vi "GPIB with VISA functions.vi"() -> ()   [LabVIEW 2020]
doc: "This example requires NI-488.2 and NI-VISA to be installed on the system. The example shows how to communicate with a GPIB instrument using VISA reads, writes, and formatting functions on the returned data. This example will work using an NI Instrument Simulator or other instrument that has similar behavior."
uses:
  <vilib>/Utility/file.llb/Write Delimited Spreadsheet (DBL).vi
  <vilib>/Analysis/NI_AALBase.lvlib
panel:
  out "Acquisition Progress":u8(slide) scale=0.0..100.0
  out "Instrument ID Response":string
  out "Current Time":timestamp
  out "XY Graph":cluster{timestamp[], dbl[]}(graph)
  out "Status Window":string
  out "Tstamp Array":timestamp[](array[timestamp])
  out "FILE WRITE":bool
  out "FILE OPEN":bool
  out "VISA OPEN":bool
  out "SAMPLE":bool
  out "Output Timestamp":timestamp[](array[timestamp])
  in  "Cancel Plot Button":bool caption="Plot Button"
  in  "EXIT":bool caption="Plot Button"
  out "Histogram Graph":T1(graph)
  out "AVG":dbl format="%^.7e"
  out "Units Display":string="VDC"
  out "LCDString":string
  in  "Plot Button":bool
  in  "INSTRUMENT MODE":T2
  out "P-P":dbl format="%^.7e"
  out "MNIDX":i32 format="%#.0f"
  out "MIN":dbl format="%^.7e"
  out "MXIDX":i32 format="%#.0f"
  out "MAX":dbl format="%^.7e"
  out "Output Value Array":dbl[](array[numeric]) format="%^#_8e"
  out "Data Array":dbl[](array[numeric]) format="%^_9e"
  out "ET":dbl format="%<%H:%M:%S%2u>t"
  out "ERROR":bool
  out "ACTIVE CONNECTION":bool
  out "UI Title String":string="IDEwerks IEE488 DataAcquisition/Logging Module" caption="String"
  in  "SETUP PARAMETERS":T3={"Samples"=1024, "NPLC"=10.0, "Digits"=7, "Auto-Zero"="ON", "Auto-Range"="ON", "ACAL on Scan"="ENABLED", "Display"="TEST IN PROGRESS", "Fixed-Z"="OFF", "Man-Range"="OFF", "Panel Lock"="OFF", "Logging"="POST SCAN", "Export Type"=""} {"Digits" min=4 max=8}
  out "SAM":i32
  out "Waveform Chart":waveform(dbl)(graph)
  out "error out":errorcluster
  out "VAL":dbl format="%.7e"
  in  "VISA GPIB Resource":refnum<visa-resource-name>="GPIB0::22::INSTR"
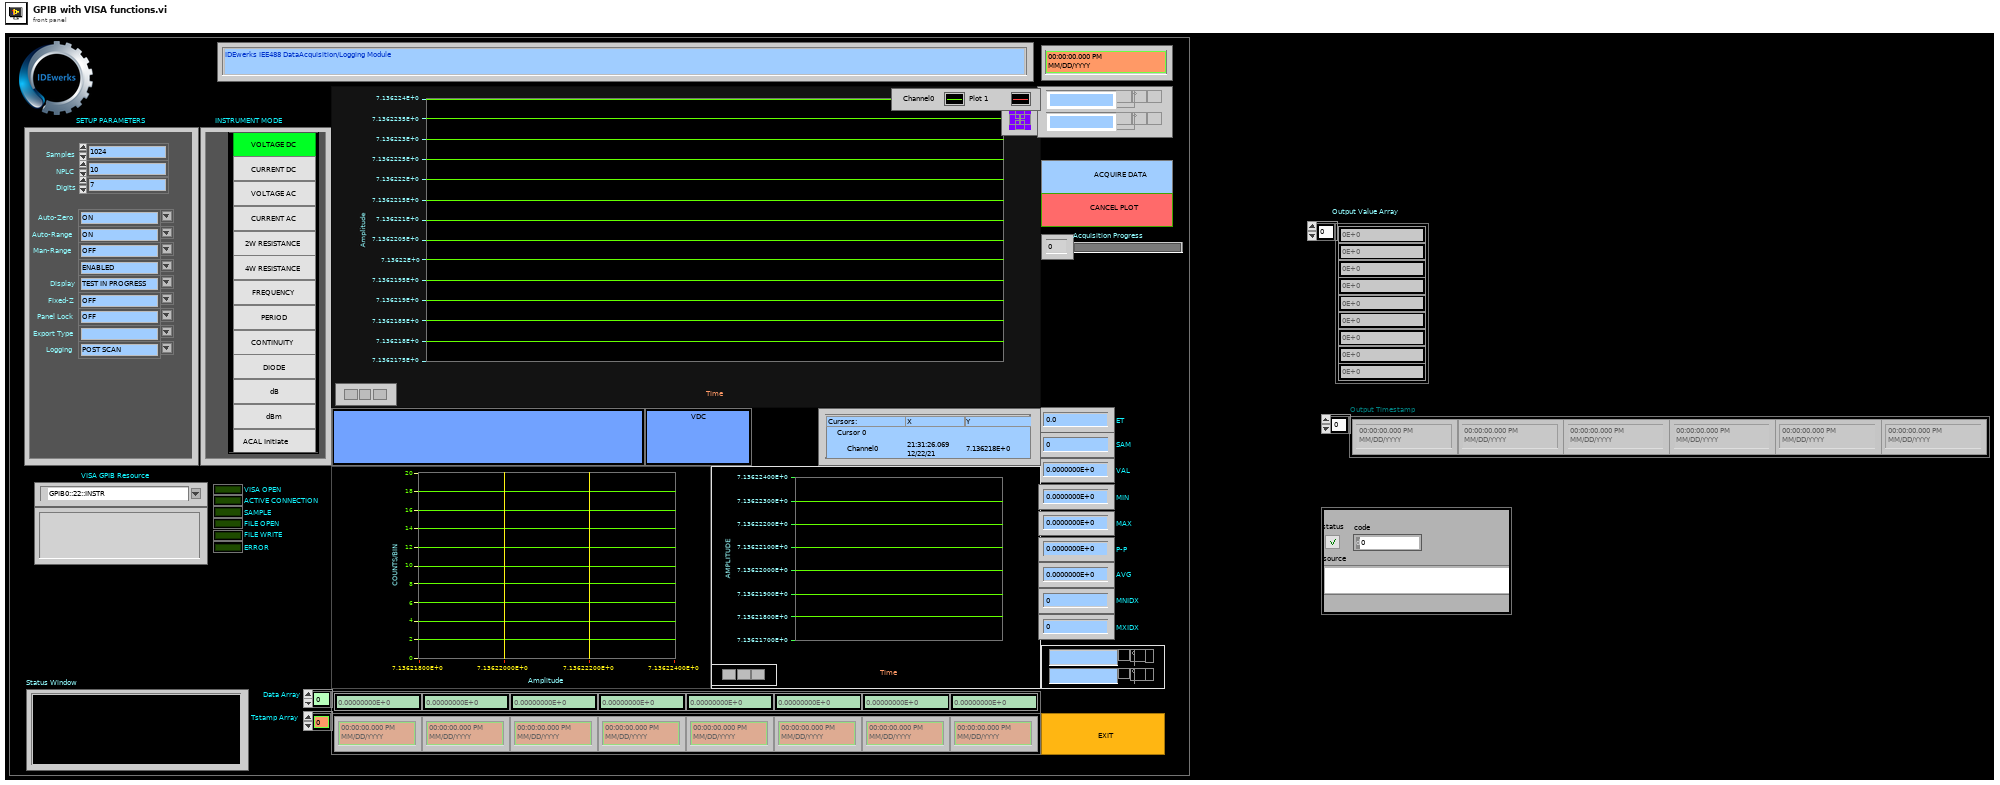
[diagram p1: front panel]
types:
  T1 = cluster{"X Values":dbl[], "Histogram: h(x)":i32[]}
  T2 = cluster{"Radio Buttons":enum32{"VDC Select Button", "IDC Select Button", "VAC Select Button", "IAC Select Button", "2WR Select Button", "4W Res Select Button", "Freq Select Button", "Period Select Button", "Continuity Select Button", "Diode Select Button", "dB Select Button", "dBm Select Button", "ACAL Select Button"}}
  T3 = cluster{"Samples":i32, "NPLC":dbl, "Digits":i32, "Auto-Zero":string, "Auto-Range":string, "ACAL on Scan":string, "Display":string, "Fixed-Z":string, "Man-Range":string, "Panel Lock":string, "Logging":string, "Export Type":string}
  T4 = enum32{"VDC Select Button", "IDC Select Button", "VAC Select Button", "IAC Select Button", "2WR Select Button", "4W Res Select Button", "Freq Select Button", "Period Select Button", "Continuity Select Button", "Diode Select Button", "dB Select Button", "dBm Select Button", "ACAL Select Button"}
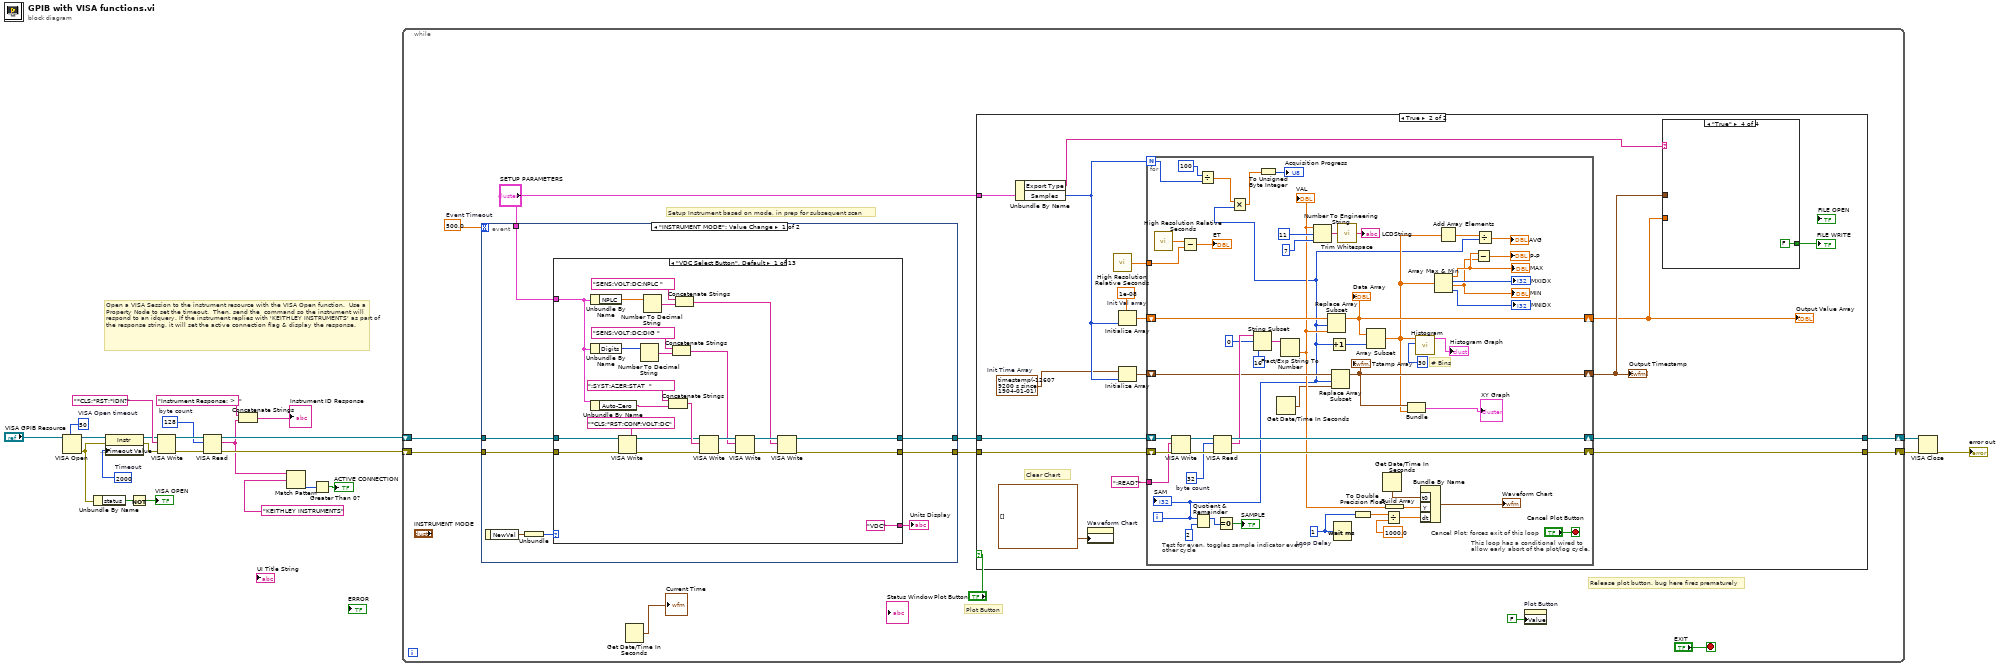
[diagram p0: block diagram]
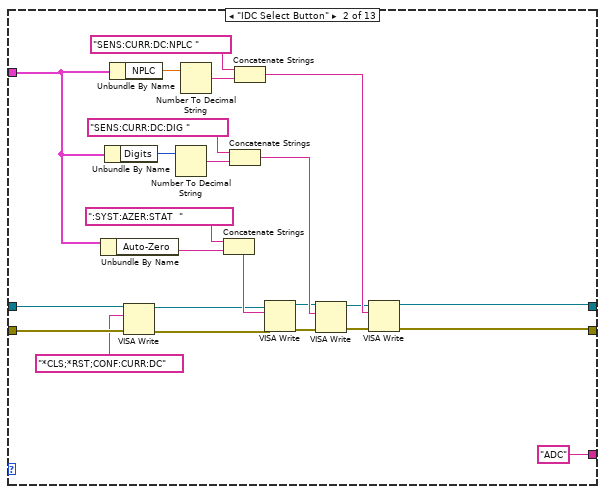
[diagram p2: hidden frame]
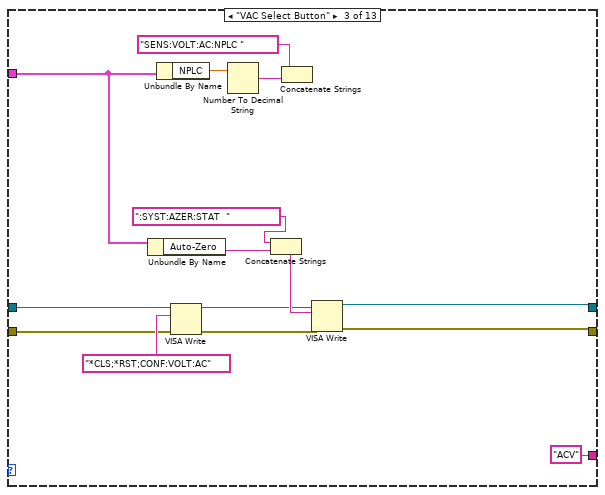
[diagram p3: hidden frame]
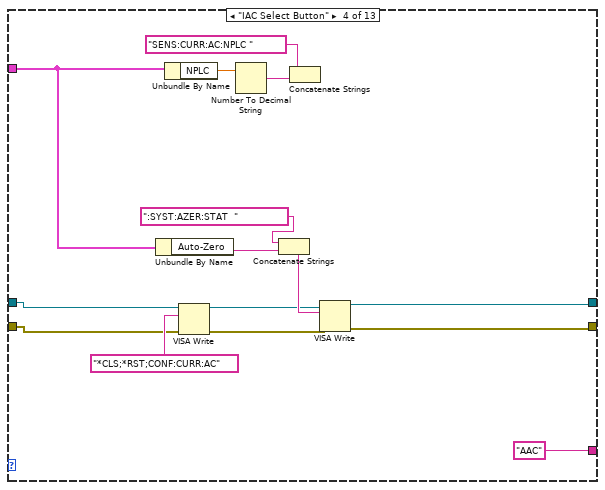
[diagram p4: hidden frame]
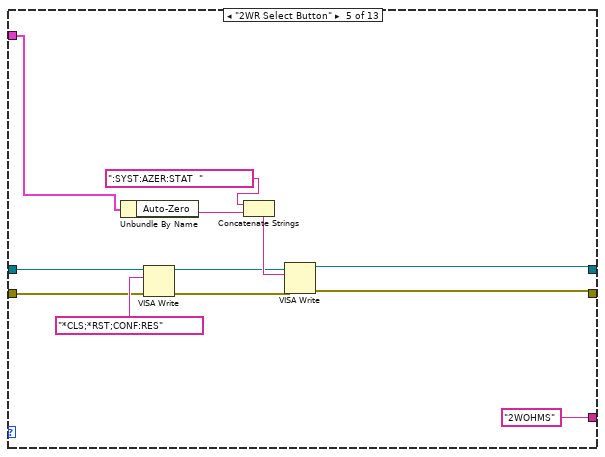
[diagram p5: hidden frame]
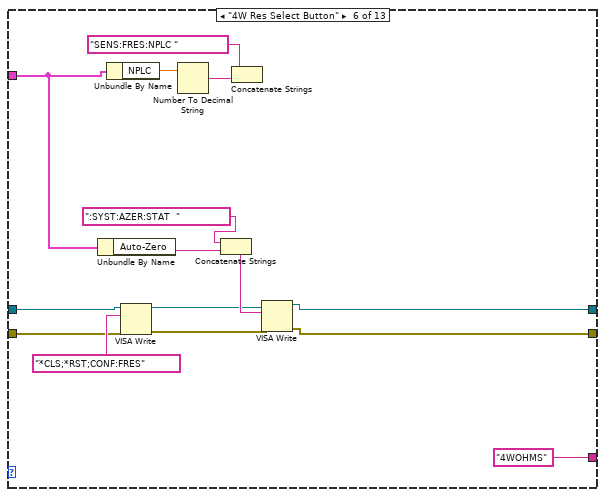
[diagram p6: hidden frame]
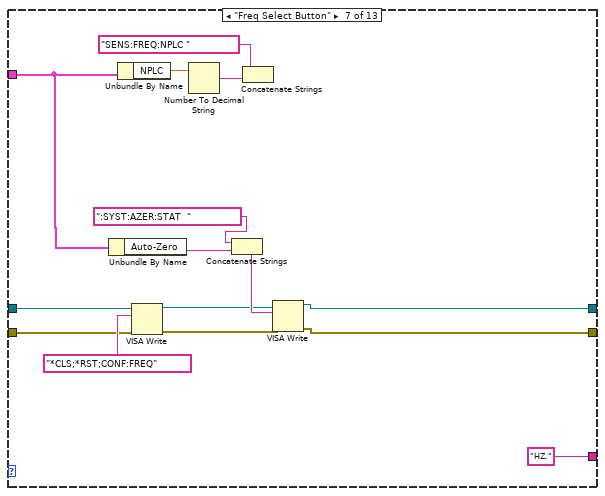
[diagram p7: hidden frame]
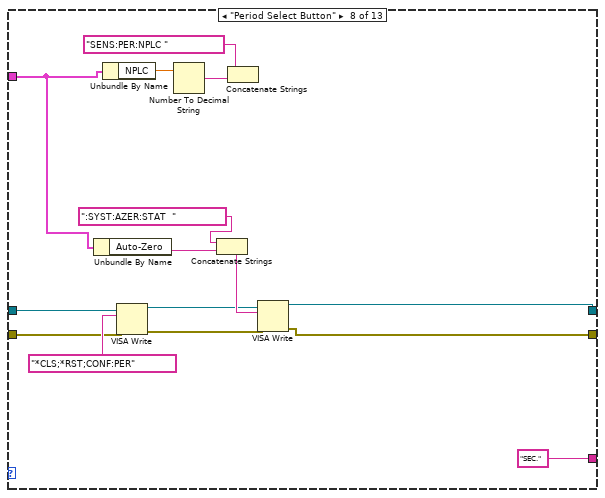
[diagram p8: hidden frame]
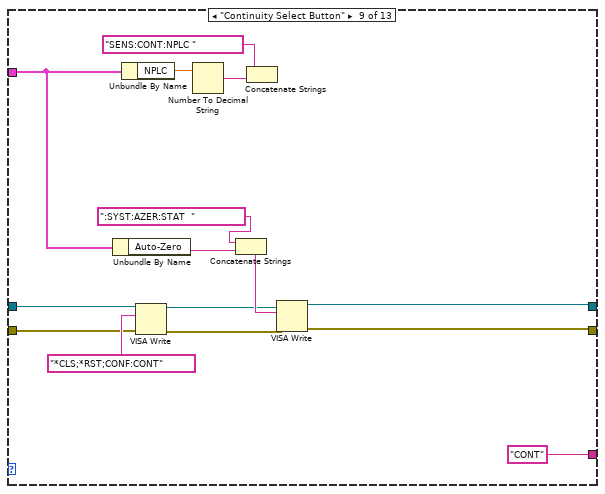
[diagram p9: hidden frame]
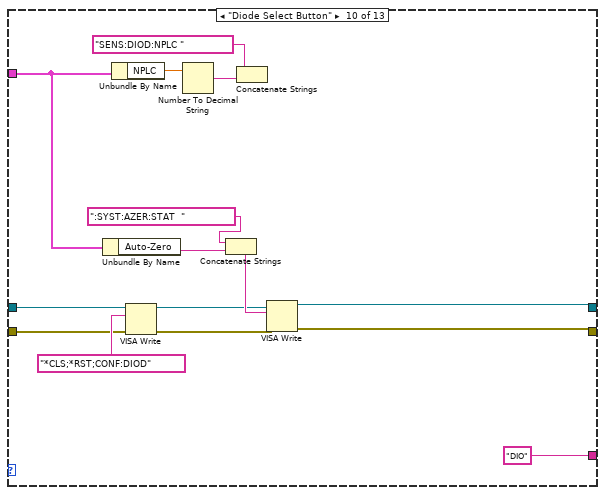
[diagram p10: hidden frame]
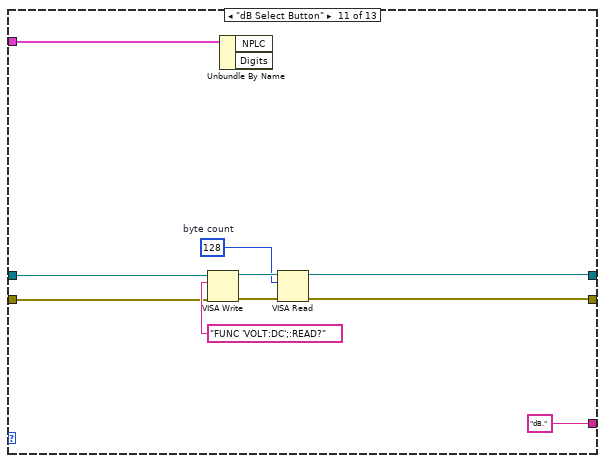
[diagram p11: hidden frame]
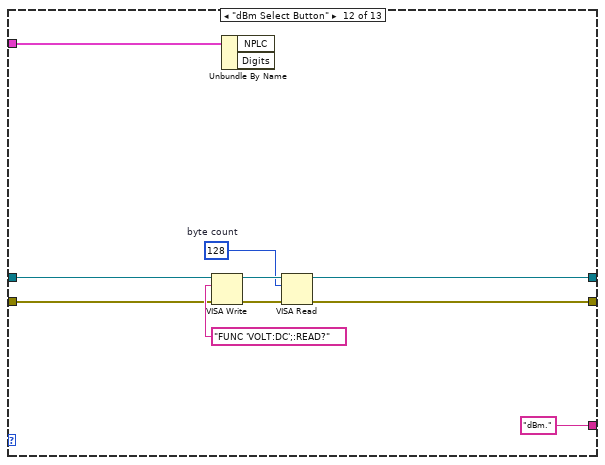
[diagram p12: hidden frame]
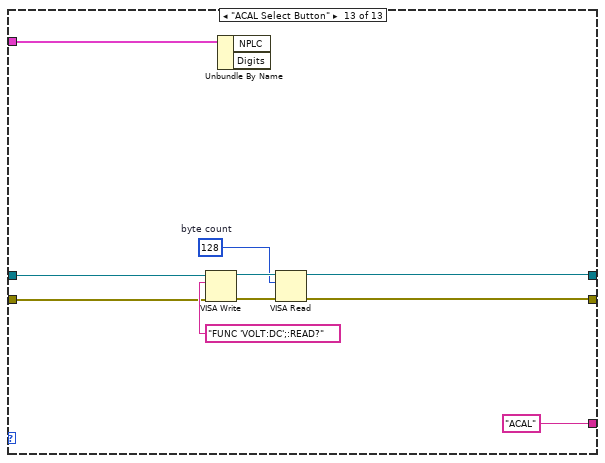
[diagram p13: hidden frame]
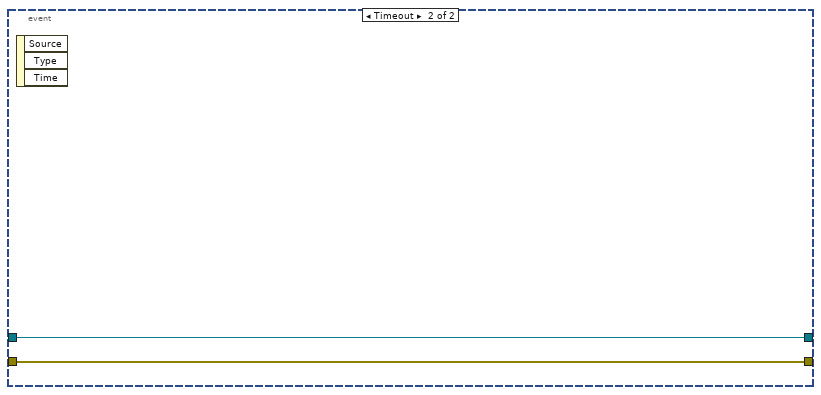
[diagram p14: hidden frame]
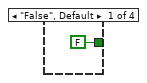
[diagram p16: hidden frame]
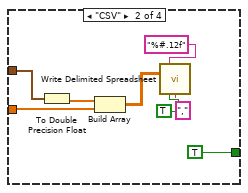
[diagram p17: hidden frame]
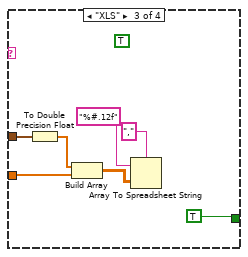
[diagram p18: hidden frame]
diagram:
  w18 = u32 128  # byte count
  w22 = u32 2000  # Timeout
  w23 = u32 50  # VISA Open timeout
  # "Open a VISA Session to the instrument resource with the VISA Open function.  Use a Property Node to set the timeout.  Then, send the  command so the instrument will respond to an idquery. If the instrument replies with 'KEITHLEY INSTRUMENTS' as part of the response string, it will set the active connection flag & display the response."
  n1 = VISA Open(timeout (0)=w23, VISA resource name="VISA GPIB Resource") -> (VISA resource name=w21:refnum<visa-resource-name>, error out=w5:errorcluster)  [unwired: 3 in]
  n2 = Unbundle By Name(w5) -> ("status"=w3:bool)
  n3 = property class="Instr"(reference=w21, error in=w5, "General Settings:Timeout Value"=w22) -> (reference out=w17:refnum<visa-resource-name>, error out=w16:errorcluster)
  n4 = Not(x=w3) -> (.not. x?=→"VISA OPEN":bool)
  n5 = VISA Write(VISA resource name=w17, write buffer="*CLS;*RST;*IDN?" ("Write Buffer"), error in (no error)=w16) -> (VISA resource name out=w24:refnum<visa-resource-name>, error out=w4:errorcluster)  [unwired: 1 out]
  n6 = VISA Read(VISA resource name=w24, byte count=w18, error in (no error)=w4) -> (VISA resource name out=w15:refnum<visa-resource-name>, read buffer=w7:string, error out=w14:errorcluster)  [unwired: 1 out]
  n7 = Concatenate Strings("Instrument Response: >  " ("Inst Response UI string constant"), w7) -> (→"Instrument ID Response":string)
  n8 = Match Pattern(string=w7, regular expression="KEITHLEY INSTRUMENTS") -> (offset past match=w6:i32)  [unwired: 1 in, 3 out]
  n9 = Greater Than 0?(x=w6) -> (x > 0?=→"ACTIVE CONNECTION":bool)
  n10 = while {
    shift-right: [w35] -> w12
    shift-left: w15 -> [w34]
    shift-right: [w36] -> w13
    shift-left: w14 -> [w33]
    stop <- "EXIT" stop-if-true
    w28 = 500.0  # Event Timeout
    # "Release plot button, bug here fires prematurely"
    # "Plot Button"
    # "Setup Instrument based on mode, in prep for subsequent scan"
    n11 = event shown="[0] \"INSTRUMENT MODE\": Value Change" {
      selector: _ -> [_ _]
      dyn-events: _ -> [_ _]
      timeout: w28 -> [_ _]
      tunnel: w34 -> [w44 w241]
      tunnel: w33 -> [w43 w240]
      tunnel: [w42 w240] -> w32
      tunnel: [w41 w241] -> w31
      tunnel: "SETUP PARAMETERS" -> [w40 _]
      event "INSTRUMENT MODE": Value Change {
        n12 = event-data() -> ("NewVal"=w39:T2)  [unwired: 1 in]
        n13 = Unbundle(w39) -> ("Radio Buttons"=w38:T4)
        n14 = case shown="\"VDC Select Button\", Default" w38 {
          tunnel: ["VDC" ("VDC string constant") "ADC" ("IDC String") "ACV" ("Inst Response UI string constant") "AAC" ("Inst Response UI string constant") "2WOHMS" ("Inst Response UI string constant") "4WOHMS" ("Inst Response UI string constant") "HZ." ("Inst Response UI string constant") "SEC." ("Inst Response UI string constant") "CONT" ("Inst Response UI string constant") "DIO" ("Inst Response UI string constant") "dB." ("Inst Response UI string constant") "dBm." ("Inst Response UI string constant") "ACAL" ("Inst Response UI string constant")] -> w37
          tunnel: w44 -> [w49 w73 w96 w112 w126 w138 w153 w168 w183 w198 w213 w223 w234]
          tunnel: w43 -> [w48 w71 w95 w111 w125 w137 w152 w167 w182 w199 w212 w222 w233]
          tunnel: [w53 w74 w93 w109 w123 w135 w150 w165 w180 w196 w210 w220 w231] -> w42
          tunnel: [w54 w75 w94 w110 w124 w136 w151 w166 w181 w197 w211 w221 w232] -> w41
          tunnel: w40 -> [w50 w83 w97 w108 w127 w139 w154 w169 w184 w195 w214 w224 w230]
          frame "VDC Select Button", Default {
            n15 = Unbundle By Name(w50) -> ("NPLC"=w59:dbl)
            n16 = Unbundle By Name(w50) -> ("Digits"=w64:i32)
            n17 = Unbundle By Name(w50) -> ("Auto-Zero"=w66:string)
            n18 = VISA Write(VISA resource name=w49, write buffer="*CLS;*RST;CONF:VOLT:DC" ("Write Buffer"), error in (no error)=w48) -> (VISA resource name out=w47:refnum<visa-resource-name>, error out=w46:errorcluster)  [unwired: 1 out]
            n19 = Number To Decimal String(number=w64) -> (decimal integer string=w63:string)  [unwired: 1 in]
            n20 = Number To Decimal String(number=w59) -> (decimal integer string=w60:string)  [unwired: 1 in]
            n21 = Concatenate Strings(":SYST:AZER:STAT  " ("Write Buffer"), w66) -> (w65:string)
            n22 = Concatenate Strings("SENS:VOLT:DC:DIG " ("Write Buffer"), w63) -> (w52:string)
            n23 = Concatenate Strings("SENS:VOLT:DC:NPLC " ("Write Buffer"), w60) -> (w51:string)
            n24 = VISA Write(VISA resource name=w47, write buffer=w65, error in (no error)=w46) -> (VISA resource name out=w56:refnum<visa-resource-name>, error out=w55:errorcluster)  [unwired: 1 out]
            n25 = VISA Write(VISA resource name=w56, write buffer=w52, error in (no error)=w55) -> (VISA resource name out=w57:refnum<visa-resource-name>, error out=w58:errorcluster)  [unwired: 1 out]
            n26 = VISA Write(VISA resource name=w57, write buffer=w51, error in (no error)=w58) -> (VISA resource name out=w54:refnum<visa-resource-name>, error out=w53:errorcluster)  [unwired: 1 out]
          }
          frame "IDC Select Button" {
            n27 = Unbundle By Name(w83) -> ("Auto-Zero"=w90:string)
            n28 = Unbundle By Name(w83) -> ("Digits"=w89:i32)
            n29 = Unbundle By Name(w83) -> ("NPLC"=w84:dbl)
            n30 = VISA Write(VISA resource name=w73, write buffer="*CLS;*RST;CONF:CURR:DC" ("Write Buffer"), error in (no error)=w71) -> (VISA resource name out=w72:refnum<visa-resource-name>, error out=w70:errorcluster)  [unwired: 1 out]
            n31 = Number To Decimal String(number=w89) -> (decimal integer string=w88:string)  [unwired: 1 in]
            n32 = Number To Decimal String(number=w84) -> (decimal integer string=w85:string)  [unwired: 1 in]
            n33 = Concatenate Strings(":SYST:AZER:STAT  " ("Write Buffer"), w90) -> (w80:string)
            n34 = Concatenate Strings("SENS:CURR:DC:DIG " ("Write Buffer"), w88) -> (w81:string)
            n35 = Concatenate Strings("SENS:CURR:DC:NPLC " ("Write Buffer"), w85) -> (w82:string)
            n36 = VISA Write(VISA resource name=w72, write buffer=w80, error in (no error)=w70) -> (VISA resource name out=w79:refnum<visa-resource-name>, error out=w76:errorcluster)  [unwired: 1 out]
            n37 = VISA Write(VISA resource name=w79, write buffer=w81, error in (no error)=w76) -> (VISA resource name out=w78:refnum<visa-resource-name>, error out=w77:errorcluster)  [unwired: 1 out]
            n38 = VISA Write(VISA resource name=w78, write buffer=w82, error in (no error)=w77) -> (VISA resource name out=w75:refnum<visa-resource-name>, error out=w74:errorcluster)  [unwired: 1 out]
          }
          frame "VAC Select Button" {
            n39 = Unbundle By Name(w97) -> ("Auto-Zero"=w106:string)
            n40 = Unbundle By Name(w97) -> ("NPLC"=w104:dbl)
            n41 = VISA Write(VISA resource name=w96, write buffer="*CLS;*RST;CONF:VOLT:AC" ("Write Buffer"), error in (no error)=w95) -> (VISA resource name out=w102:refnum<visa-resource-name>, error out=w101:errorcluster)  [unwired: 1 out]
            n42 = Number To Decimal String(number=w104) -> (decimal integer string=w105:string)  [unwired: 1 in]
            n43 = Concatenate Strings(":SYST:AZER:STAT  " ("Write Buffer"), w106) -> (w103:string)
            n44 = Concatenate Strings("SENS:VOLT:AC:NPLC " ("Write Buffer"), w105) -> ()  [unwired: 1 out]
            n45 = VISA Write(VISA resource name=w102, write buffer=w103, error in (no error)=w101) -> (VISA resource name out=w94:refnum<visa-resource-name>, error out=w93:errorcluster)  [unwired: 1 out]
          }
          frame "IAC Select Button" {
            n46 = Unbundle By Name(w108) -> ("Auto-Zero"=w121:string)
            n47 = Unbundle By Name(w108) -> ("NPLC"=w119:dbl)
            n48 = VISA Write(VISA resource name=w112, write buffer="*CLS;*RST;CONF:CURR:AC" ("Write Buffer"), error in (no error)=w111) -> (VISA resource name out=w117:refnum<visa-resource-name>, error out=w116:errorcluster)  [unwired: 1 out]
            n49 = Number To Decimal String(number=w119) -> (decimal integer string=w120:string)  [unwired: 1 in]
            n50 = Concatenate Strings(":SYST:AZER:STAT  " ("Write Buffer"), w121) -> (w118:string)
            n51 = Concatenate Strings("SENS:CURR:AC:NPLC " ("Write Buffer"), w120) -> ()  [unwired: 1 out]
            n52 = VISA Write(VISA resource name=w117, write buffer=w118, error in (no error)=w116) -> (VISA resource name out=w110:refnum<visa-resource-name>, error out=w109:errorcluster)  [unwired: 1 out]
          }
          frame "2WR Select Button" {
            n53 = Unbundle By Name(w127) -> ("Auto-Zero"=w133:string)
            n54 = VISA Write(VISA resource name=w126, write buffer="*CLS;*RST;CONF:RES" ("Write Buffer"), error in (no error)=w125) -> (VISA resource name out=w131:refnum<visa-resource-name>, error out=w130:errorcluster)  [unwired: 1 out]
            n55 = Concatenate Strings(":SYST:AZER:STAT  " ("Write Buffer"), w133) -> (w132:string)
            n56 = VISA Write(VISA resource name=w131, write buffer=w132, error in (no error)=w130) -> (VISA resource name out=w124:refnum<visa-resource-name>, error out=w123:errorcluster)  [unwired: 1 out]
          }
          frame "4W Res Select Button" {
            n57 = Unbundle By Name(w139) -> ("Auto-Zero"=w148:string)
            n58 = Unbundle By Name(w139) -> ("NPLC"=w146:dbl)
            n59 = VISA Write(VISA resource name=w138, write buffer="*CLS;*RST;CONF:FRES" ("Write Buffer"), error in (no error)=w137) -> (VISA resource name out=w144:refnum<visa-resource-name>, error out=w143:errorcluster)  [unwired: 1 out]
            n60 = Number To Decimal String(number=w146) -> (decimal integer string=w147:string)  [unwired: 1 in]
            n61 = Concatenate Strings(":SYST:AZER:STAT  " ("Write Buffer"), w148) -> (w145:string)
            n62 = Concatenate Strings("SENS:FRES:NPLC " ("Write Buffer"), w147) -> ()  [unwired: 1 out]
            n63 = VISA Write(VISA resource name=w144, write buffer=w145, error in (no error)=w143) -> (VISA resource name out=w136:refnum<visa-resource-name>, error out=w135:errorcluster)  [unwired: 1 out]
          }
          frame "Freq Select Button" {
            n64 = Unbundle By Name(w154) -> ("Auto-Zero"=w163:string)
            n65 = Unbundle By Name(w154) -> ("NPLC"=w161:dbl)
            n66 = VISA Write(VISA resource name=w153, write buffer="*CLS;*RST;CONF:FREQ" ("Write Buffer"), error in (no error)=w152) -> (VISA resource name out=w159:refnum<visa-resource-name>, error out=w158:errorcluster)  [unwired: 1 out]
            n67 = Number To Decimal String(number=w161) -> (decimal integer string=w162:string)  [unwired: 1 in]
            n68 = Concatenate Strings(":SYST:AZER:STAT  " ("Write Buffer"), w163) -> (w160:string)
            n69 = Concatenate Strings("SENS:FREQ:NPLC " ("Write Buffer"), w162) -> ()  [unwired: 1 out]
            n70 = VISA Write(VISA resource name=w159, write buffer=w160, error in (no error)=w158) -> (VISA resource name out=w151:refnum<visa-resource-name>, error out=w150:errorcluster)  [unwired: 1 out]
          }
          frame "Period Select Button" {
            n71 = Unbundle By Name(w169) -> ("Auto-Zero"=w178:string)
            n72 = Unbundle By Name(w169) -> ("NPLC"=w176:dbl)
            n73 = VISA Write(VISA resource name=w168, write buffer="*CLS;*RST;CONF:PER" ("Write Buffer"), error in (no error)=w167) -> (VISA resource name out=w174:refnum<visa-resource-name>, error out=w173:errorcluster)  [unwired: 1 out]
            n74 = Number To Decimal String(number=w176) -> (decimal integer string=w177:string)  [unwired: 1 in]
            n75 = Concatenate Strings(":SYST:AZER:STAT  " ("Write Buffer"), w178) -> (w175:string)
            n76 = Concatenate Strings("SENS:PER:NPLC " ("Write Buffer"), w177) -> ()  [unwired: 1 out]
            n77 = VISA Write(VISA resource name=w174, write buffer=w175, error in (no error)=w173) -> (VISA resource name out=w166:refnum<visa-resource-name>, error out=w165:errorcluster)  [unwired: 1 out]
          }
          frame "Continuity Select Button" {
            n78 = Unbundle By Name(w184) -> ("Auto-Zero"=w193:string)
            n79 = Unbundle By Name(w184) -> ("NPLC"=w191:dbl)
            n80 = VISA Write(VISA resource name=w183, write buffer="*CLS;*RST;CONF:CONT" ("Write Buffer"), error in (no error)=w182) -> (VISA resource name out=w189:refnum<visa-resource-name>, error out=w188:errorcluster)  [unwired: 1 out]
            n81 = Number To Decimal String(number=w191) -> (decimal integer string=w192:string)  [unwired: 1 in]
            n82 = Concatenate Strings(":SYST:AZER:STAT  " ("Write Buffer"), w193) -> (w190:string)
            n83 = Concatenate Strings("SENS:CONT:NPLC " ("Write Buffer"), w192) -> ()  [unwired: 1 out]
            n84 = VISA Write(VISA resource name=w189, write buffer=w190, error in (no error)=w188) -> (VISA resource name out=w181:refnum<visa-resource-name>, error out=w180:errorcluster)  [unwired: 1 out]
          }
          frame "Diode Select Button" {
            n85 = Unbundle By Name(w195) -> ("Auto-Zero"=w208:string)
            n86 = Unbundle By Name(w195) -> ("NPLC"=w206:dbl)
            n87 = VISA Write(VISA resource name=w198, write buffer="*CLS;*RST;CONF:DIOD" ("Write Buffer"), error in (no error)=w199) -> (VISA resource name out=w204:refnum<visa-resource-name>, error out=w203:errorcluster)  [unwired: 1 out]
            n88 = Number To Decimal String(number=w206) -> (decimal integer string=w207:string)  [unwired: 1 in]
            n89 = Concatenate Strings(":SYST:AZER:STAT  " ("Write Buffer"), w208) -> (w205:string)
            n90 = Concatenate Strings("SENS:DIOD:NPLC " ("Write Buffer"), w207) -> ()  [unwired: 1 out]
            n91 = VISA Write(VISA resource name=w204, write buffer=w205, error in (no error)=w203) -> (VISA resource name out=w197:refnum<visa-resource-name>, error out=w196:errorcluster)  [unwired: 1 out]
          }
          frame "dB Select Button" {
            w216 = u32 128  # byte count
            n92 = VISA Write(VISA resource name=w213, write buffer="FUNC 'VOLT:DC';:READ?" ("Write Buffer"), error in (no error)=w212) -> (VISA resource name out=w217:refnum<visa-resource-name>, error out=w218:errorcluster)  [unwired: 1 out]
            n93 = Unbundle By Name(w214) -> ()  [unwired: 2 out]
            n94 = VISA Read(VISA resource name=w217, byte count=w216, error in (no error)=w218) -> (VISA resource name out=w211:refnum<visa-resource-name>, error out=w210:errorcluster)  [unwired: 2 out]
          }
          frame "dBm Select Button" {
            w226 = u32 128  # byte count
            n95 = VISA Write(VISA resource name=w223, write buffer="FUNC 'VOLT:DC';:READ?" ("Write Buffer"), error in (no error)=w222) -> (VISA resource name out=w227:refnum<visa-resource-name>, error out=w228:errorcluster)  [unwired: 1 out]
            n96 = Unbundle By Name(w224) -> ()  [unwired: 2 out]
            n97 = VISA Read(VISA resource name=w227, byte count=w226, error in (no error)=w228) -> (VISA resource name out=w221:refnum<visa-resource-name>, error out=w220:errorcluster)  [unwired: 2 out]
          }
          frame "ACAL Select Button" {
            w236 = u32 128  # byte count
            n98 = VISA Write(VISA resource name=w234, write buffer="FUNC 'VOLT:DC';:READ?" ("Write Buffer"), error in (no error)=w233) -> (VISA resource name out=w237:refnum<visa-resource-name>, error out=w238:errorcluster)  [unwired: 1 out]
            n99 = Unbundle By Name(w230) -> ()  [unwired: 2 out]
            n100 = VISA Read(VISA resource name=w237, byte count=w236, error in (no error)=w238) -> (VISA resource name out=w232:refnum<visa-resource-name>, error out=w231:errorcluster)  [unwired: 2 out]
          }
        }
        "Units Display" <- w37
      }
      event Timeout {
        n101 = event-data() -> ()  [unwired: 1 in, 3 out]
      }
    }
    n102 = Get Date/Time In Seconds() -> (seconds since 1Jan1904=→"Current Time":timestamp)
    n103 = case shown="True" "Plot Button" {
      tunnel: w31 -> [w243 w260]
      tunnel: w32 -> [w242 w259]
      tunnel: [w242 w258] -> w36
      tunnel: [w243 w257] -> w35
      tunnel: "SETUP PARAMETERS" -> [_ w250]
      frame False {
      }
      frame True {
        w254 = 1e-08  # Init Val array
        w248 = timestamp(-126079199.5371399 s since 1904-01-01)  # Init Time Array
        # "Clear Chart"
        n104 = Unbundle By Name(w250) -> ("Export Type"=w247:string, "Samples"=w249:i32)
        n105 = property on="Waveform Chart" class="WFChart (strict)"("History Data"=waveform(dbl)[] []) -> ()  [unwired: 2 in, 2 out]
        n106 = call <vilib>:"High Resolution Relative Seconds.vi"() -> ("relative seconds"=w256:dbl)
        n107 = Initialize Array(w254, w249) -> (w253:dbl[])
        n108 = Initialize Array(w248, w249) -> (w255:timestamp[])
        n109 = for {
          N: w249 -> [w283]
          shift-right: [w325] -> w257
          shift-left: w260 -> [w331]
          shift-right: [w327] -> w258
          shift-left: w259 -> [w329]
          tunnel: w256 -> [w314]
          shift-right: [w286] -> w246
          shift-left: w255 -> [w311]
          shift-right: [w288] -> w245
          shift-left: w253 -> [w310]
          tunnel: ":READ?" ("Write Buffer") -> [w300]
          i -> [w280]
          stop <- "Cancel Plot Button" stop-if-true
          w318 = u32 1  # Loop Delay
          w326 = u32 32  # byte count
          # "Test for even, toggles sample indicator every other cycle"
          # "Cancel Plot; forces exit of this loop"
          # "This loop has a conditional wired to allow early abort of the plot/log cycle."
          # "# Bins"
          n110 = call <vilib>:"High Resolution Relative Seconds.vi"() -> ("relative seconds"=w313:dbl)
          n111 = VISA Write(VISA resource name=w331, write buffer=w300, error in (no error)=w329) -> (VISA resource name out=w330:refnum<visa-resource-name>, error out=w328:errorcluster)  [unwired: 1 out]
          n112 = Subtract(x=w313, y=w314) -> (x-y=→"ET":dbl)
          n113 = Quotient & Remainder(x=w280, y=2) -> (x-y*floor(x/y)=w294:i32)  [unwired: 1 out]
          n114 = Divide(x=100 ("y"), y=w283) -> (x/y=w281:dbl)
          n115 = VISA Read(VISA resource name=w330, byte count=w326, error in (no error)=w328) -> (VISA resource name out=w325:refnum<visa-resource-name>, read buffer=w323:string, error out=w327:errorcluster)  [unwired: 1 out]
          n116 = Equal To 0?(x=w294) -> (x = 0?=→"SAMPLE":bool)
          n117 = Multiply(x=w281, y=w280) -> (x*y=w278:dbl)
          n118 = String Subset(string=w323, offset (0)=0, length (rest)=16 ("length (rest)")) -> (substring=w324:string)
          n119 = To Unsigned Byte Integer(number=w278) -> (unsigned 8bit integer=→"Acquisition Progress":u8)
          n120 = Get Date/Time In Seconds() -> (seconds since 1Jan1904=w290:timestamp)
          n121 = Fract/Exp String To Number(string=w324) -> (number=w291:dbl)  [unwired: 3 in, 1 out]
          "VAL" <- w291
          n122 = Number To Engineering String(2:7 ("offset (0)"), 3:11 ("offset (0)"), 4:w291) -> (0:w301:string)  [unwired: 1 in]
          n123 = Replace Array Subset(array=w310, new element=w291, index=w280) -> (w288:dbl[])
          "Data Array" <- w288
          n124 = Increment(x=w280) -> (x+1=w284:i32)
          n125 = Replace Array Subset(array=w311, new element=w290, index=w280) -> (w286:timestamp[])
          "Tstamp Array" <- w286
          n126 = Wait (ms)(milliseconds to wait=w318) -> ()  [unwired: 1 out]
          n127 = call <vilib>:"Trim Whitespace.vi"("string"=w301) -> ("trimmed string"=→"LCDString":string)  [unwired: 1 in]
          n128 = To Double Precision Float(number=w318) -> (double precision float=w319:dbl)
          n129 = Array Subset(array=w288, length=w284) -> (w285:dbl[])  [unwired: 1 in]
          n130 = Get Date/Time In Seconds() -> (seconds since 1Jan1904=w315:timestamp)
          n131 = Divide(x=w319, y=1000.0) -> (x/y=w316:dbl)
          n132 = Build Array(w291) -> (w317:dbl[])
          n133 = Bundle(w286, w285) -> (→"XY Graph":cluster{timestamp[], dbl[]})  [unwired: 1 in]
          n134 = call <vilib>:"Histogram.vi"("intervals"=30, "X"=w285) -> ("Histogram Graph"=→"Histogram Graph":T1)  [unwired: 6 in, 3 out]
          n135 = Bundle By Name("t0"=w315, "Y"=w317, "dt"=w316) -> (→"Waveform Chart":waveform(dbl))  [unwired: 1 in]
          n136 = Array Max & Min(array=w285) -> (max value=w307:dbl, max index (indices)=→"MXIDX":i32, min value=w306:dbl, min index (indices)=→"MNIDX":i32)
          "MAX" <- w307
          "MIN" <- w306
          n137 = Add Array Elements(numeric array=w285) -> (sum=w299:dbl)
          n138 = Subtract(x=w307, y=w306) -> (x-y=→"P-P":dbl)
          n139 = Divide(x=w299, y=w280) -> (x/y=→"AVG":dbl)
          "SAM" <- w280
        }
        "Output Value Array" <- w245
        "Output Timestamp" <- w246
        n140 = case shown="\"True\"" w247 {
          tunnel: w246 -> [_ w267 w275 _]
          tunnel: w245 -> [_ w266 w274 _]
          tunnel: [FALSE ("FILE WRITE") TRUE ("FILE WRITE") TRUE ("FILE WRITE") FALSE ("FILE WRITE")] -> w244
          frame "False", Default {
          }
          frame "CSV" {
            n141 = To Double Precision Float(number=w267) -> (double precision float=w269:dbl[])
            n142 = Build Array(w269, w266) -> (w268:dbl[][])
            n143 = call-poly <vilib>:"Write Delimited Spreadsheet.vi"("format (%.3f)"="%#.12f", "2D data"=w268, "transpose? (no:F)"=TRUE, "delimiter (\\t)"="," ("delimiter (\\t)")) -> ()  [unwired: 10 in, 2 out]
          }
          frame "XLS" {
            (unwired) TRUE ("Reset")
            n144 = To Double Precision Float(number=w275) -> (double precision float=w276:dbl[])
            n145 = Build Array(w276, w274) -> (w273:dbl[][])
            n146 = Array To Spreadsheet String(delimiter (Tab)=",", array=w273, 3:"%#.12f" ("format string")) -> ()  [unwired: 1 out]
          }
          frame "True" {
          }
        }
        "FILE WRITE" <- w244
      }
    }
    n147 = property on="Plot Button" class="Bool (strict)"("Value"=FALSE) -> ()  [unwired: 2 in, 2 out]
  }
  n148 = VISA Close(VISA resource name=w12, error in (no error)=w13) -> (error out=→"error out":errorcluster)
